vi "Contoh read write digital output 1 line.vi"() -> ()   [LabVIEW 2020]
uses:
  <vilib>/DAQmx/read.llb/DAQmx Read (Digital Bool 1Line 1Point).vi
  <vilib>/DAQmx/write.llb/DAQmx Write (Digital Bool 1Line 1Point).vi
  <vilib>/DAQmx/create/channels.llb/DAQmx Create Channel (DO-Digital Output).vi
  <vilib>/DAQmx/create/channels.llb/DAQmx Create Channel (DI-Digital Input).vi
  <vilib>/DAQmx/miscellaneous.llb/DAQmx Fill In Error Info.vi
panel:
  out "Boolean 2":bool
  in  "DAQmx Physical Channel 2":tag
  in  "stop":bool
  in  "Boolean":bool
  in  "DAQmx Physical Channel":tag
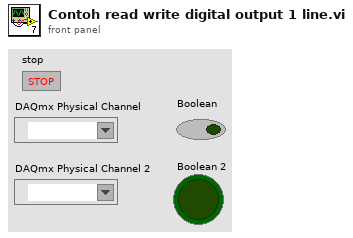
[diagram p1: front panel]
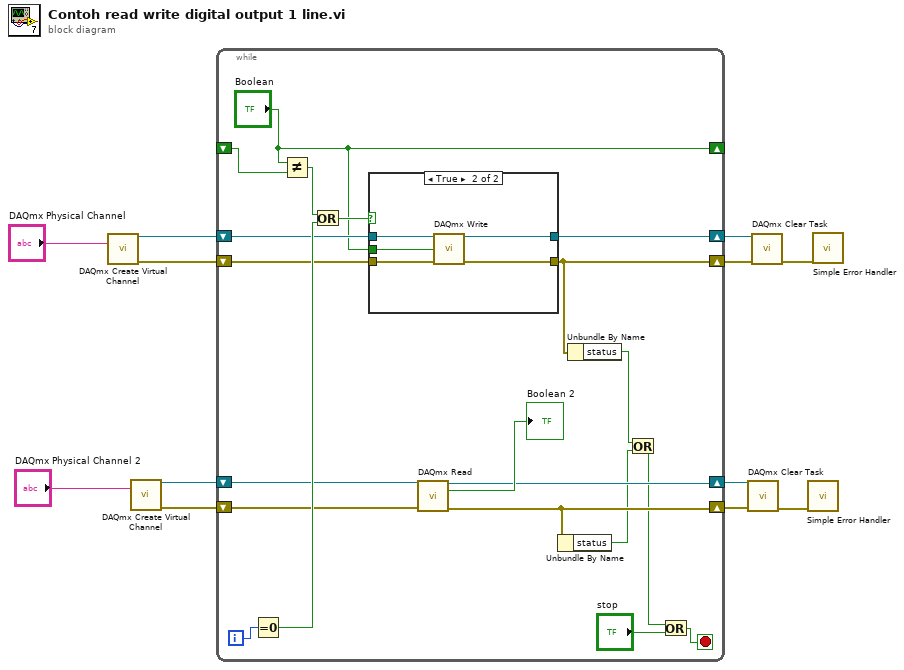
[diagram p0: block diagram]
diagram:
  n1 = call-poly <vilib>:"DAQmx Create Virtual Channel.vi"("lines"="DAQmx Physical Channel") -> ("task out"=w11:refnum<k21>, "error out"=w10:errorcluster)  [unwired: 13 in]
  n2 = call-poly <vilib>:"DAQmx Create Virtual Channel.vi"("lines"="DAQmx Physical Channel 2") -> ("task out"=w5:refnum<k21>, "error out"=w4:errorcluster)  [unwired: 13 in]
  n3 = while {
    shift-right: ["Boolean"] -> _
    shift-left: _ -> [w31]
    shift-right: [w21] -> w8
    shift-left: w10 -> [w26]
    shift-right: [w24] -> w9
    shift-left: w11 -> [w27]
    shift-right: [w17] -> w2
    shift-left: w5 -> [w20]
    shift-right: [w16] -> w1
    shift-left: w4 -> [w19]
    i -> [w32]
    stop <- w23 stop-if-true
    n4 = Equal To 0?(x=w32) -> (x = 0?=w29:bool)
    n5 = Not Equal?(x="Boolean", y=w31) -> (x != y?=w30:bool)
    n6 = Or(x=w30, y=w29) -> (x .or. y?=w28:bool)
    n7 = case shown="True" w28 {
      tunnel: w27 -> [w34 w39]
      tunnel: w26 -> [w33 w38]
      tunnel: "Boolean" -> [_ w37]
      tunnel: [w34 w36] -> w24
      tunnel: [w33 w35] -> w21
      frame False {
      }
      frame True {
        n8 = call-poly <vilib>:"DAQmx Write.vi"("task/channels in"=w39, "data"=w37, "error in"=w38) -> ("task out"=w36:refnum<k21>, "error out"=w35:errorcluster)  [unwired: 10 in, 1 out]
      }
    }
    n9 = call-poly <vilib>:"DAQmx Read.vi"("task/channels in"=w20, "error in"=w19) -> ("task out"=w17:refnum<k21>, "data"=→"Boolean 2":bool, "error out"=w16:errorcluster)  [unwired: 11 in]
    n10 = Unbundle By Name(w16) -> ("status"=w14:bool)
    n11 = Unbundle By Name "Unbundle By Name"(w21) -> ("status"=w15:bool)
    n12 = Or(x=w15, y=w14) -> (x .or. y?=w13:bool)
    n13 = Or(x=w13, y="stop") -> (x .or. y?=w23:bool)
  }
  n14 = call <vilib>:"DAQmx Clear Task.vi"("task in"=w2, "error in"=w1) -> ("error out"=w3:errorcluster)  [unwired: 13 in]
  n15 = call <vilib>:"DAQmx Clear Task.vi"("task in"=w9, "error in"=w8) -> ("error out"=w7:errorcluster)  [unwired: 13 in]
  n16 = call <vilib>:"Simple Error Handler.vi"("error in (no error)"=w3) -> ()  [unwired: 4 in, 5 out]
  n17 = call <vilib>:"Simple Error Handler.vi"("error in (no error)"=w7) -> ()  [unwired: 4 in, 5 out]
